vi "Get Unvisited Neighbors.vi"(7 "Unvisited":bool[][][](array[boolean]), 11 "Current Point":i32[](array[numeric])) -> (3 "Unvisited Neighbors":cluster{"X":i32, "Y":i32, "Dir":i32}[](array[cluster]))   [LabVIEW 2021]
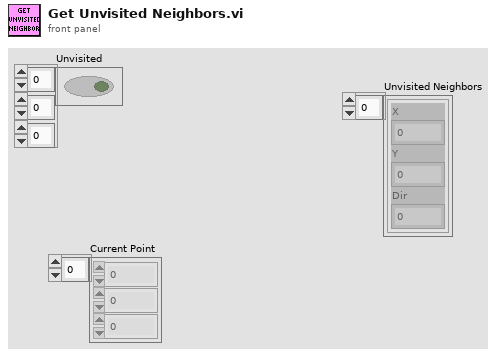
[diagram p1: front panel]
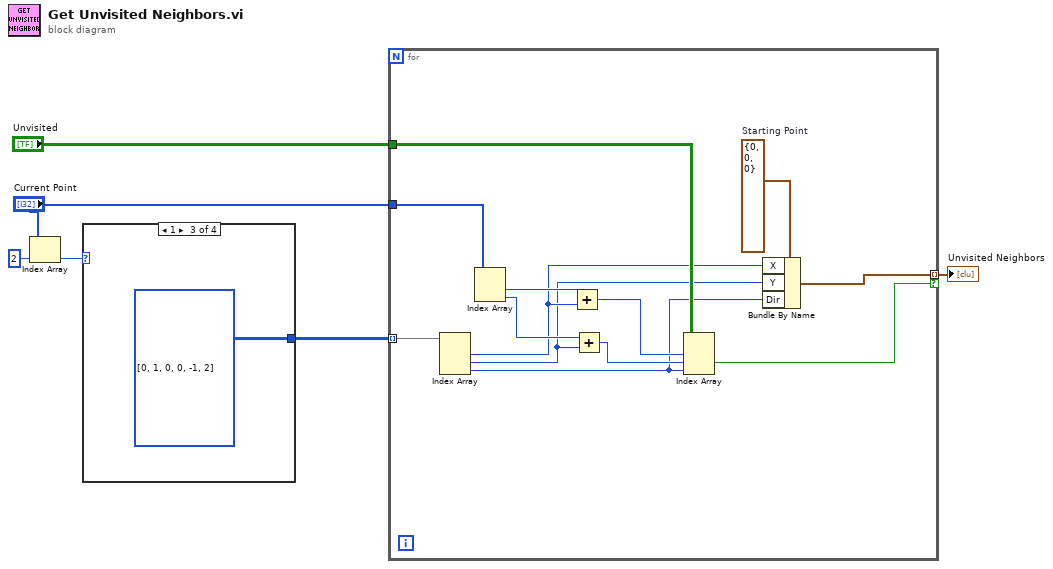
[diagram p0: block diagram]
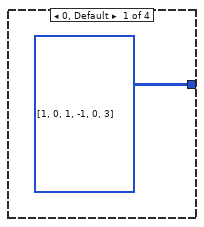
[diagram p2: hidden frame]
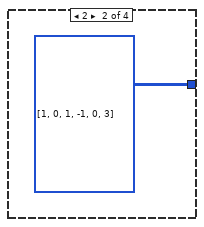
[diagram p3: hidden frame]
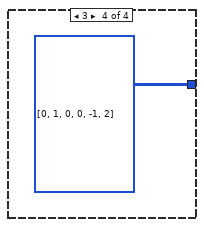
[diagram p4: hidden frame]
diagram:
  n1 = Index Array(array="Current Point", index=2) -> (element=w1:i32)
  n2 = case shown="1" w1 {
    tunnel: [i32[][] [[1, 0, 1], [-1, 0, 3]] i32[][] [[1, 0, 1], [-1, 0, 3]] i32[][] [[0, 1, 0], [0, -1, 2]] i32[][] [[0, 1, 0], [0, -1, 2]]] -> w2
    frame 0, Default {
    }
    frame 2 {
    }
    frame 1 {
    }
    frame 3 {
    }
  }
  n3 = for {
    tunnel: "Current Point" -> [w19]
    tunnel: "Unvisited" -> [w23]
    tunnel: [w21] -> w5 mode=indexing if=w20
    tunnel: w2 -> [w18] mode=indexing
    w22 = cluster{"X":i32, "Y":i32, "Dir":i32} {"X"=0, "Y"=0, "Dir"=0}  # Starting Point
    n4 = Index Array(array=w18) -> (element #1=w13:i32, element #2=w12:i32, element #3=w11:i32)  [unwired: 3 in]
    n5 = Index Array(array=w19) -> (element #1=w17:i32, element #2=w15:i32)  [unwired: 2 in]
    n6 = Add(x=w17, y=w13) -> (x+y=w16:i32)
    n7 = Add(x=w15, y=w12) -> (x+y=w14:i32)
    n8 = Index Array(array=w23, index (dim 0)=w16, index (dim 1)=w14, index (dim 2)=w11) -> (element=w20:bool)
    n9 = Bundle By Name(cluster=w22, "X"=w13, "Y"=w12, "Dir"=w11) -> (w21:cluster{"X":i32, "Y":i32, "Dir":i32})
  }
  "Unvisited Neighbors" <- w5
